vi "Add Result.vi"(8 "error in (no error)":errorcluster, 10 "Result.lvclass":refnum<class "Result.lvclass">, 11 "Report in":refnum<class "Report.lvclass">) -> (0 "error out":errorcluster, 3 "Report out":refnum<class "Report.lvclass">)   [LabVIEW 2015, in "Report.lvclass"]
doc: "This VI takes a result and saves it to a local object for writing to disk later."
uses:
  Report.lvclass
  Result/Result.lvclass
  Report.lvclass/Report.ctl
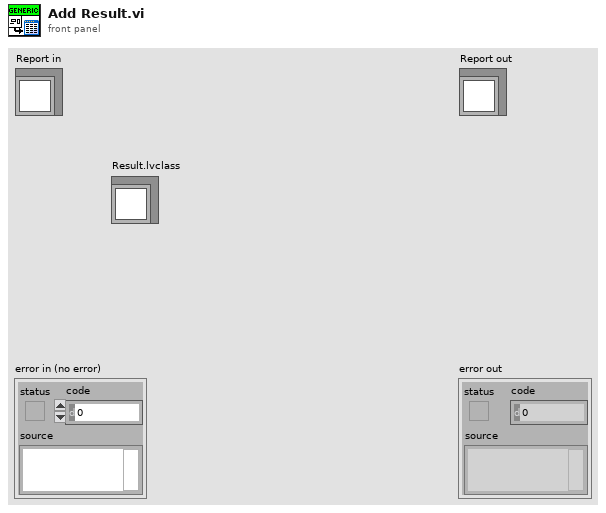
[diagram p1: front panel]
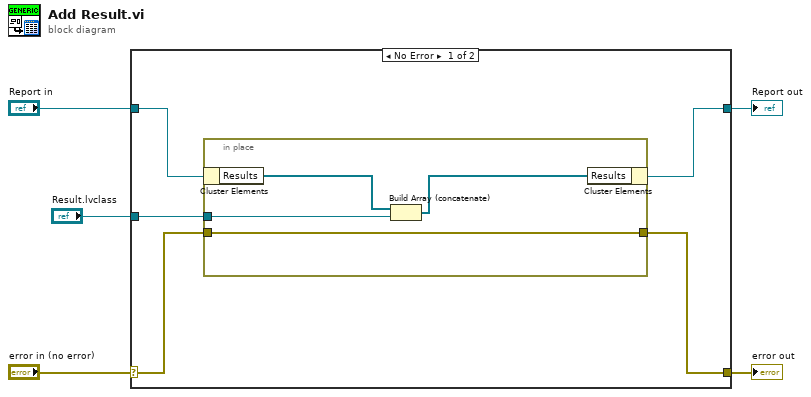
[diagram p0: block diagram]
diagram:
  n1 = case shown="No Error" "error in (no error)" {
    selector: "error in (no error)" -> [w9 w16]
    tunnel: [w8 w16] -> w4
    tunnel: [w7 w15] -> w2
    tunnel: "Report in" -> [w10 w15]
    tunnel: "Result.lvclass" -> [w6 _]
    frame No Error {
      n2 = in-place {
        in-place-border: w9 -> [w11]
        in-place-border: w6 -> [w14]
        in-place-border: [w11] -> w8
        n3 = in-place-cluster #1(w10) -> ("Results"=w13:refnum<class "Result.lvclass">[])
        n4 = Build Array (concatenate)(w13, w14) -> (w12:refnum<class "Result.lvclass">[])
        n5 = in-place-cluster #1("Results"=w12) -> (w7:refnum<class "Report.lvclass">)
      }
    }
    frame Error {
    }
  }
  "error out" <- w4
  "Report out" <- w2
